vi "U3 DAC_Kevin_MFC.vi"() -> ()   [LabVIEW 2016]
uses:
  <vilib>/Utility/file.llb/Read From Spreadsheet File (DBL).vi
  <vilib>/measure/NI_MABase.lvlib
panel:
  in  "DAC0_type":enum16{"functional", "fixed", "read"}(ring)
  out "Array Size":i32
  out "Udate Array from File":sgl[](array[numeric])
  out "Waveform Chart":dbl(graph)
  in  "DAC0_fixed":dbl step=0.1 format="%.4f"
  out "Error Message":string
  out "error out":errorcluster
  in  "DAC1&DACB_fixed":dbl step=0.1 format="%.4f"
  in  "Update Interval (ms)":u32=20
  out "Error":string
  in  "Function":u16(ring) items=["Sine Wave", "Triangle Wave", "Square Wave", "Sawtooth Wave"]
  in  "Min Voltage":dbl=0.5 min=0.0 max=5.0 step=0.1 format="%.2f"
  in  "Max Voltage":dbl=4.5 min=0.0 max=5.0 step=0.1 format="%.2f"
  in  "Frequency (Hz)":dbl=1.0 step=0.1 format="%.3f"
  in  "Stop":bool
  # "Updates DAC0 at the specified update interval in order to build time series waveforms.  The\nupdate interval is set to 20 ms by default, but can be set lower based on the execution times\ndiscussed in Section 3.1 of the U3 User's Guide.  Uses the first found U3.\n\nWith a software timed application such as this, you might be able to reduce timing jitter (caused\nby the operating system) by increasing the priority of this process (labview.exe) in Windows\nTask Manager."
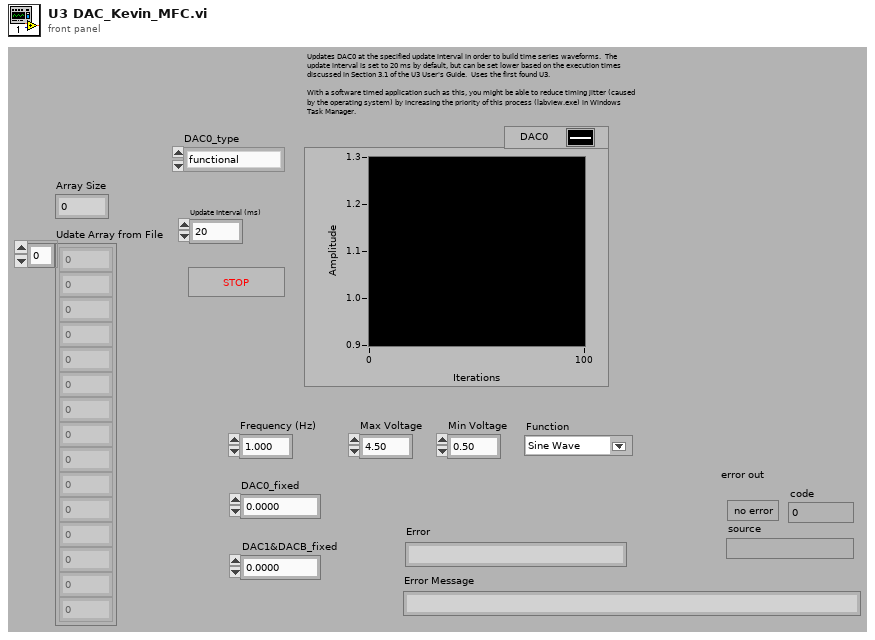
[diagram p1: front panel]
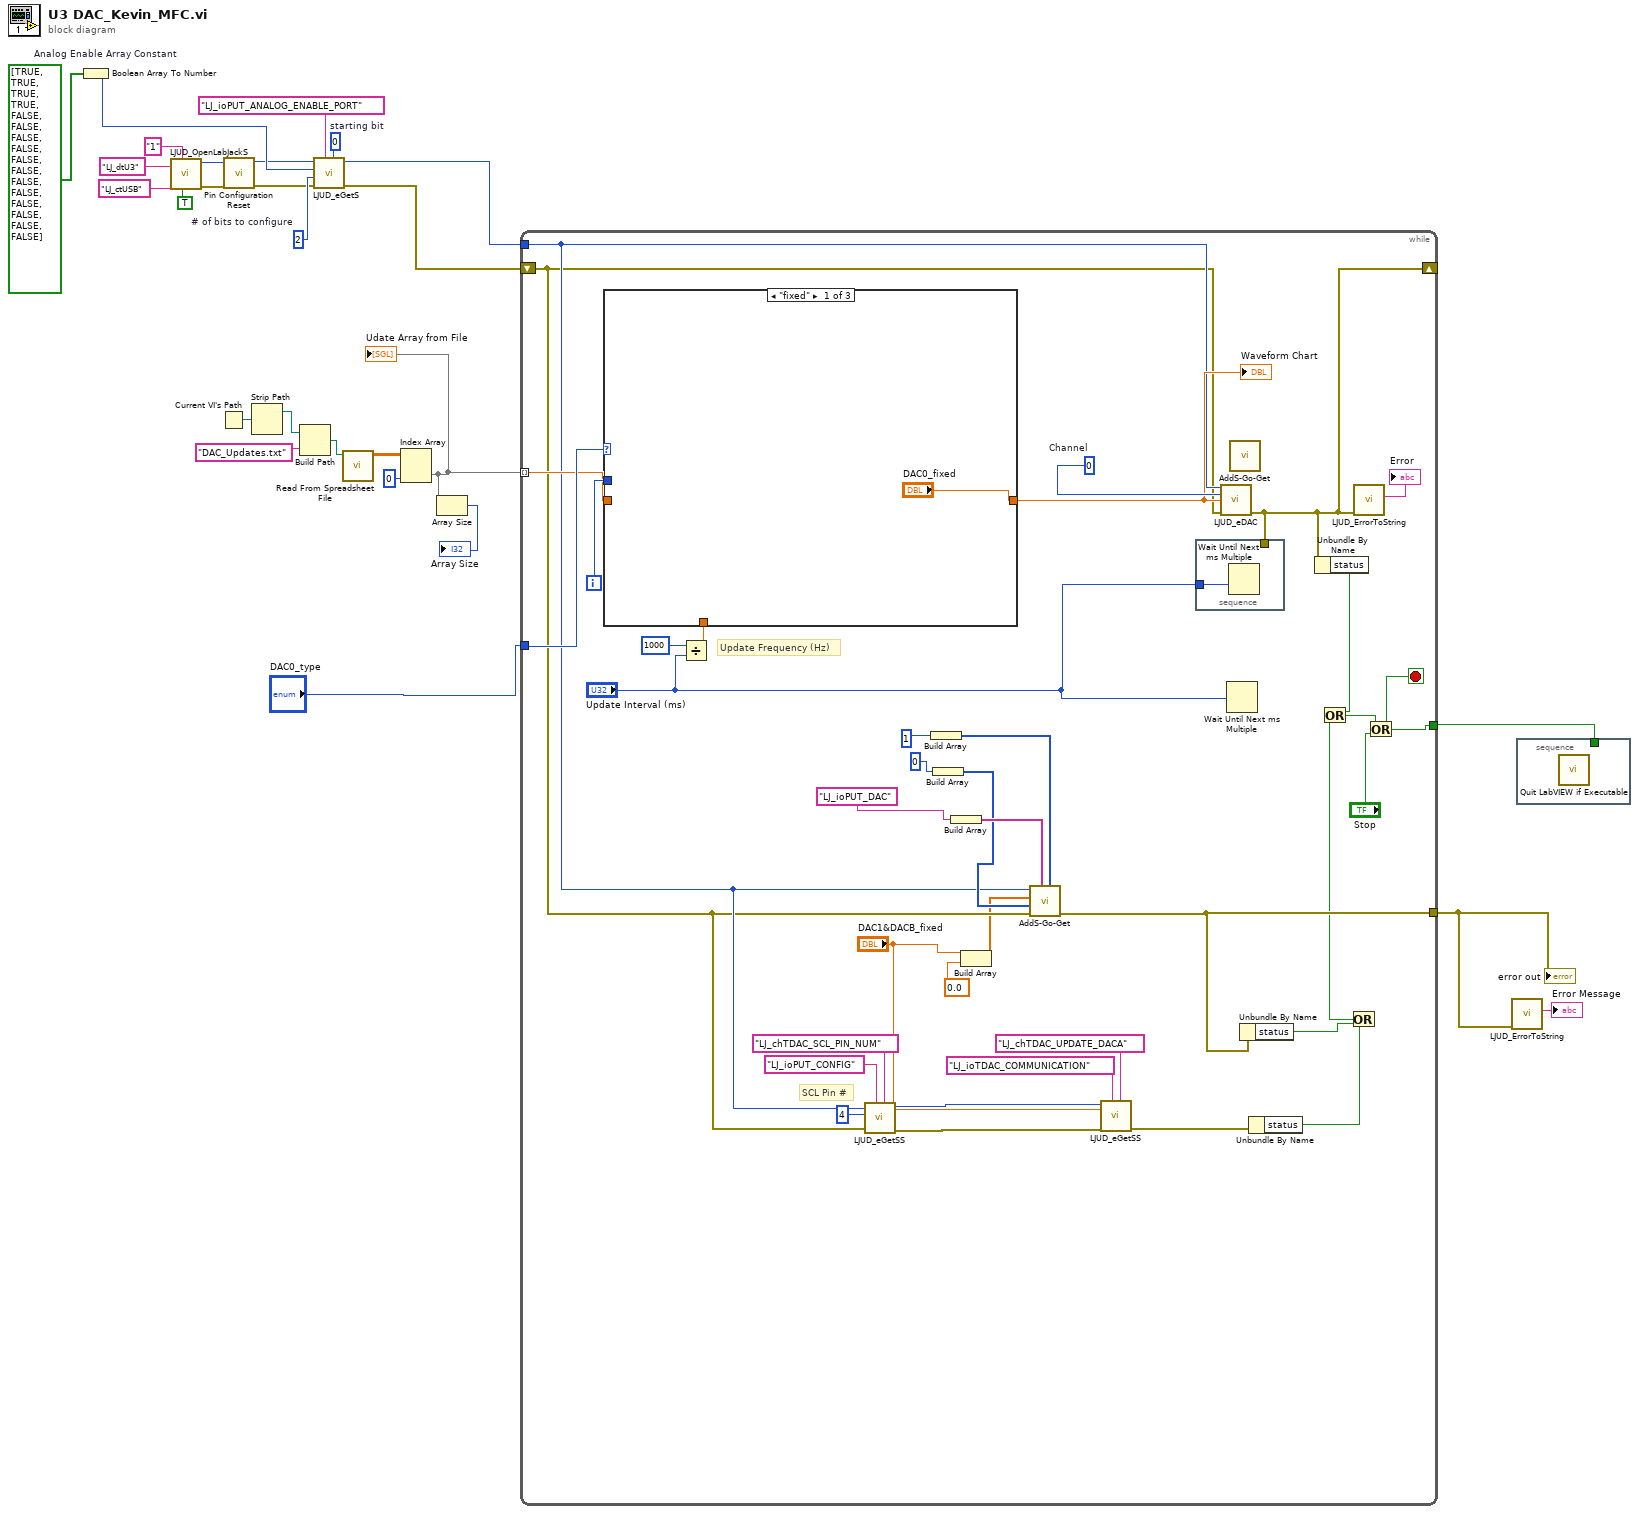
[diagram p0: block diagram]
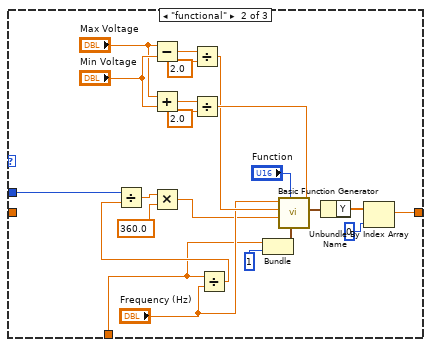
[diagram p2: hidden frame]
diagram:
  w6 = 2  # # of bits to configure
  w8 = 0  # starting bit
  w9 = bool[] [TRUE, TRUE, TRUE, TRUE, FALSE, FALSE, FALSE, FALSE, FALSE, FALSE, FALSE, FALSE, FALSE, FALSE, FALSE, FALSE]  # Analog Enable Array Constant
  n1 = Boolean Array To Number(Boolean array=w9) -> (number=w5:u32)
  n2 = call "LJUD_OpenLabJackS.vi"("FirstFound"=TRUE, "Address"="1" ("DeviceType"), "ConnectionType"="LJ_ctUSB", "DeviceType"="LJ_dtU3") -> ("error out"=w10:errorcluster, "Handle"=w11:i32)  [unwired: 5 in, 1 out]
  n3 = Current VI's Path() -> (path=w19:path)
  n4 = call "Pin Configuration Reset.vi"("error in"=w10, "Handle In"=w11) -> ("error out"=w3:errorcluster, "Handle Out"=w4:i32)  [unwired: 8 in]
  n5 = Strip Path(path=w19) -> (stripped path=w18:path)  [unwired: 1 out]
  n6 = Build Path(base path=w18, name or relative path="DAC_Updates.txt" ("file path (dialog if empty)")) -> (appended path=w20:path)
  n7 = call "LJUD_eGetS.vi"("Channel"=w8, "IOType"="LJ_ioPUT_ANALOG_ENABLE_PORT", "error in"=w3, "x1"=w6, "Value Write"=w5, "Handle In"=w4) -> ("error out"=w1:errorcluster, "Handle Out"=w2:i32)  [unwired: 3 in, 1 out]
  n8 = call-poly <vilib>:"Read From Spreadsheet File.vi"("file path (dialog if empty)"=w20) -> ("all rows"=w24:dbl[][])  [unwired: 6 in, 4 out]
  n9 = Index Array(array=w24, index (col)=0 ("disabled index (col)")) -> (element=w17:dbl[])  [unwired: 1 in]
  "Udate Array from File" <- w17
  n10 = Array Size(array=w17) -> (size(s)=→"Array Size":i32)
  n11 = while {
    tunnel: w2 -> [w39]
    shift-left: w1 -> [w38]
    shift-right: [w60] -> _
    tunnel: [w46] -> w27
    tunnel: [w49] -> w25
    tunnel: "DAC0_type" -> [w44]
    tunnel: w17 -> [w43] mode=indexing
    i -> [w64]
    stop <- w46 stop-if-true
    w61 = 0  # Channel
    # "SCL Pin #"
    # "Update Frequency (Hz)"
    n12 = Divide(x=u32 1000, y="Update Interval (ms)") -> (x/y=w58:dbl)
    n13 = case shown="\"fixed\"" w44 {
      tunnel: w64 -> [_ w87 _]
      tunnel: ["DAC0_fixed" w67 w88] -> w45
      tunnel: w58 -> [_ w66 _]
      tunnel: w43 -> [_ _ w88]
      frame "fixed" {
      }
      frame "functional" {
        n14 = Subtract(x="Max Voltage", y="Min Voltage") -> (x-y=w84:dbl)
        n15 = Add(x="Max Voltage", y="Min Voltage") -> (x+y=w81:dbl)
        n16 = Divide(x=w84, y=2.0) -> (x/y=w76:dbl)
        n17 = Divide(x=w81, y=2.0) -> (x/y=w77:dbl)
        n18 = Divide(x=w66, y="Frequency (Hz)") -> (x/y=w86:dbl)
        n19 = Divide(x=w87, y=w86) -> (x/y=w85:dbl)
        n20 = Multiply(x=w85, y=360.0) -> (x*y=w73:dbl)
        n21 = Bundle(w66, 1) -> (w71:cluster{dbl, i32})  [unwired: 1 in]
        n22 = call <vilib>:"Basic Function Generator.vi"("offset"=w77, "sampling info"=w71, "signal type"="Function", "phase"=w73, "amplitude"=w76, "frequency"="Frequency (Hz)") -> ("signal out"=w70:waveform(dbl))  [unwired: 3 in, 2 out]
        n23 = Unbundle By Name(w70) -> ("Y"=w69:dbl[])
        n24 = Index Array(array=w69, index=0 ("Index")) -> (element=w67:dbl)
      }
      frame "read" {
      }
    }
    "Waveform Chart" <- w45
    n25 = call "LJUD_eGetSS.vi"("Channel"="LJ_chTDAC_SCL_PIN_NUM", "IOType"="LJ_ioPUT_CONFIG", "error in"=w38, "Value Write"=4, "Handle In"=w39) -> ("error out"=w29:errorcluster, "Handle Out"=w30:i32)  [unwired: 4 in, 1 out]
    n26 = Build Array(1) -> (w56:i32[])
    n27 = Build Array(0) -> (w51:i32[])
    n28 = Build Array("LJ_ioPUT_DAC" ("IOType")) -> (w57:string[])
    n29 = Build Array("DAC1&DACB_fixed", 0.0 ("Input Element")) -> (w37:dbl[])
    n30 = call "AddS-Go-Get.vi"("Channels"=w56, "IOTypes"=w57, "error in"=w38, "x1"=w51, "Values Write"=w37, "Handle In"=w39) -> ("error out"=w49:errorcluster)  [unwired: 3 in, 2 out]
    n31 = call "LJUD_eGetSS.vi"("Channel"="LJ_chTDAC_UPDATE_DACA", "IOType"="LJ_ioTDAC_COMMUNICATION", "error in"=w29, "Value Write"="DAC1&DACB_fixed", "Handle In"=w30) -> ("error out"=w31:errorcluster)  [unwired: 4 in, 2 out]
    n32 = call "LJUD_eDAC.vi"("Handle In"=w39, "Channel"=w61, "Voltage"=w45, "error in"=w38) -> ("error out"=w60:errorcluster)  [unwired: 10 in, 1 out]
    n33 = stacked-sequence {
      tunnel: "Update Interval (ms)" -> [w89]
      tunnel: w60 -> [_]
      frame #0 {
        n34 = Wait Until Next ms Multiple(millisecond multiple=w89) -> ()  [unwired: 1 out]
      }
    }
    n35 = Wait Until Next ms Multiple(millisecond multiple="Update Interval (ms)") -> ()  [unwired: 1 out]
    n36 = call "AddS-Go-Get.vi"() -> ()  [unwired: 9 in, 3 out]
    n37 = Unbundle By Name(w49) -> ("status"=w34:bool)
    n38 = Unbundle By Name(w31) -> ("status"=w35:bool)
    n39 = Unbundle By Name(w60) -> ("status"=w48:bool)
    n40 = Or(x=w35, y=w34) -> (x .or. y?=w36:bool)
    n41 = Or(x=w48, y=w36) -> (x .or. y?=w47:bool)
    n42 = call "LJUD_ErrorToString.vi"("error in"=w60) -> ("String"=→"Error":string)  [unwired: 10 in]
    n43 = Or(x=w47, y="Stop") -> (x .or. y?=w46:bool)
  }
  "error out" <- w25
  n44 = call "LJUD_ErrorToString.vi"("error in"=w25) -> ("String"=→"Error Message":string)  [unwired: 10 in]
  n45 = stacked-sequence {
    tunnel: w27 -> [_]
    frame #0 {
      n46 = call "Quit LabVIEW if Executable.vi"() -> ()  [unwired: 1 in]
    }
  }
